vi "Position Boolean Indicator Absolute.vi"(0 "Button Ref":refnum<vi>, 1 "Left Offset (px)":i32, 2 "Top Offste (px)":i32, 3 "Height (px)":u32, 4 "Width (px)":u32, 5 "Error In":errorcluster) -> (19 "Error Out":errorcluster)   [LabVIEW 2014]
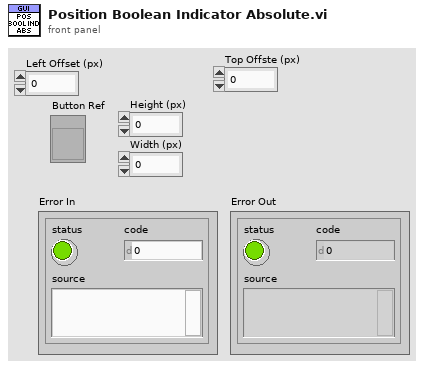
[diagram p1: front panel]
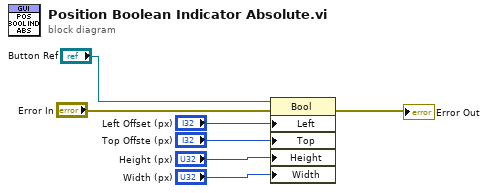
[diagram p0: block diagram]
diagram:
  n1 = property class="Bool"(reference="Button Ref", error in="Error In", "Left"="Left Offset (px)", "Top"="Top Offste (px)", "Height"="Height (px)", "Width"="Width (px)") -> (error out=→"Error Out":errorcluster)  [unwired: 1 out]
